vi "Control2Display.vi"(11 "Motor Control Cluster":T1) -> (3 "Motor Control Cluster":T1)   [LabVIEW 2021]
uses:
  TypeDef/MotorControlCluster.ctl
  controls/Status Lights.ctl
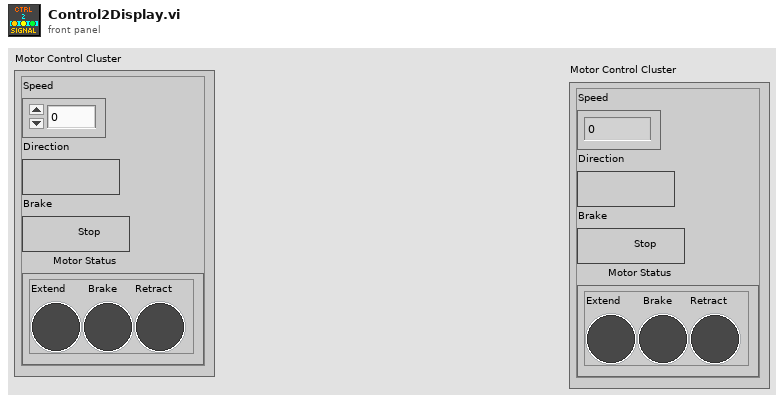
[diagram p1: front panel]
types:
  T1 = typedef "MotorControlCluster.ctl" = cluster{"Speed":dbl, "Direction":bool, "Brake":bool, "Motor Status":T2}
  T2 = typedef "Status Lights.ctl" = cluster{"Extend":bool, "Brake":bool, "Retract":bool}
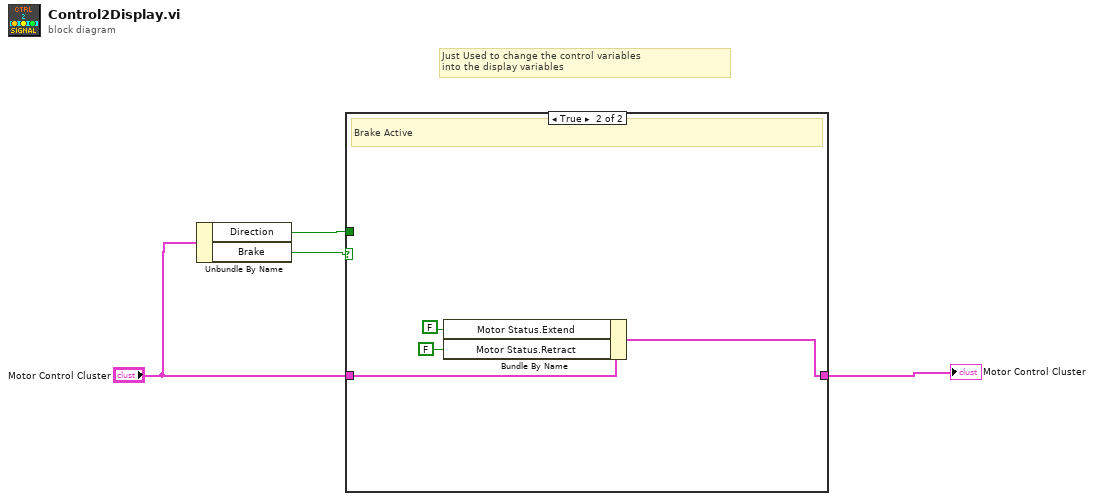
[diagram p0: block diagram]
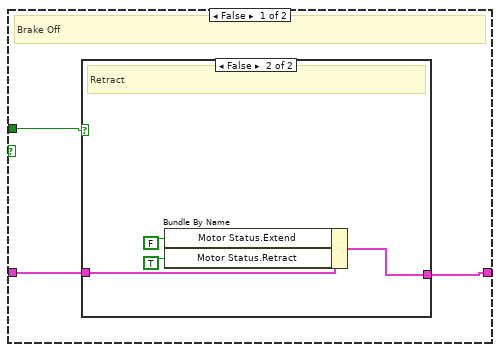
[diagram p2: hidden frame]
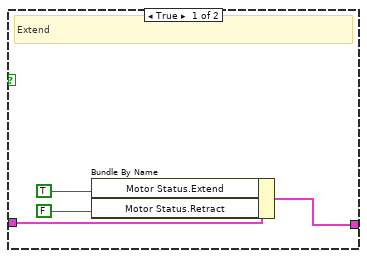
[diagram p3: hidden frame]
diagram:
  # "Just Used to change the control variables\ninto the display variables"
  n1 = Unbundle By Name("Motor Control Cluster") -> ("Direction"=w3:bool, "Brake"=w4:bool)
  n2 = case shown="True" w4 {
    tunnel: "Motor Control Cluster" -> [w7 w17]
    tunnel: [w6 w16] -> w2
    tunnel: w3 -> [w5 _]
    frame False {
      # "Brake Off"
      n3 = case shown="False" w5 {
        tunnel: w7 -> [w11 w15]
        tunnel: [w10 w14] -> w6
        frame True {
          # "Extend"
          n4 = Bundle By Name(cluster=w11, "Motor Status.Extend"=TRUE, "Motor Status.Retract"=FALSE) -> (w10:T1)
        }
        frame False {
          # "Retract"
          n5 = Bundle By Name(cluster=w15, "Motor Status.Extend"=FALSE, "Motor Status.Retract"=TRUE) -> (w14:T1)
        }
      }
    }
    frame True {
      # "Brake Active"
      n6 = Bundle By Name(cluster=w17, "Motor Status.Extend"=FALSE, "Motor Status.Retract"=FALSE) -> (w16:T1)
    }
  }
  "Motor Control Cluster" <- w2
